vi "StringInit.vi"(10 "accOUTNAME":string, 11 "dimension size":i32) -> (3 "result string":string)   [LabVIEW 2018]
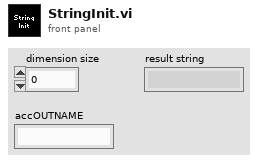
[diagram p1: front panel]
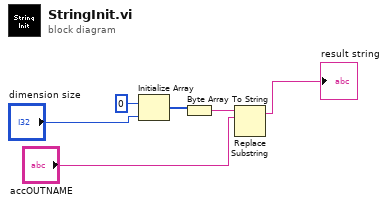
[diagram p0: block diagram]
diagram:
  n1 = Initialize Array(u8 0 ("element"), "dimension size") -> (w3:u8[])
  n2 = Byte Array To String(unsigned byte array=w3) -> (string=w2:string)
  n3 = Replace Substring(4:"accOUTNAME", 5:w2) -> (1:→"result string":string)  [unwired: 2 in, 1 out]
